vi "Dictionary ( Variant ).vi"() -> ()   [LabVIEW 2013]
panel:
  out "values":variant[](array[variant])
  out "names":string[](array[string])
  out "variant out":variant
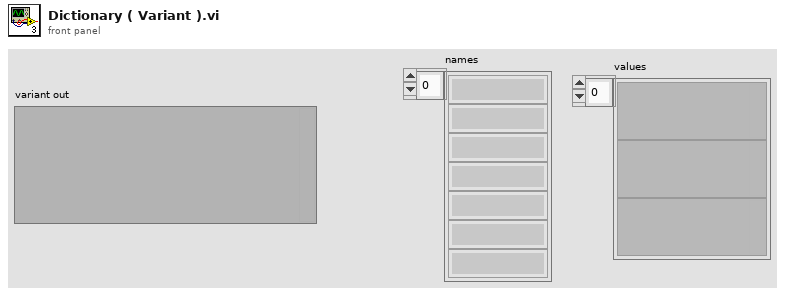
[diagram p1: front panel]
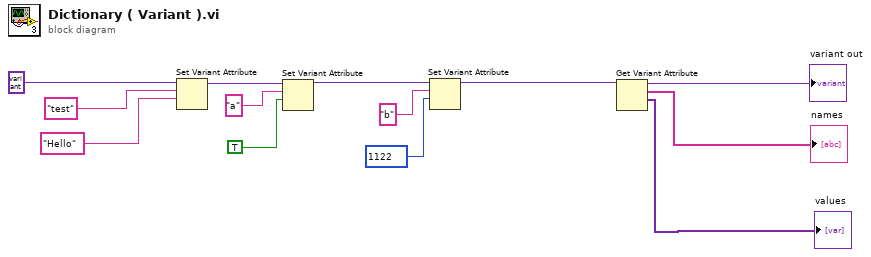
[diagram p0: block diagram]
diagram:
  n1 = Set Variant Attribute(Variant=variant ("variant"), name="test", value="Hello" ("name")) -> (Variant out=w8:variant)  [unwired: 1 in, 2 out]
  n2 = Set Variant Attribute(Variant=w8, name="a", value=TRUE) -> (Variant out=w4:variant)  [unwired: 1 in, 2 out]
  n3 = Set Variant Attribute(Variant=w4, name="b", value=1122) -> (Variant out=w3:variant)  [unwired: 1 in, 2 out]
  n4 = Get Variant Attribute(Variant=w3) -> (duplicate Variant=→"variant out":variant, names=→"names":string[], values=→"values":variant[])  [unwired: 3 in, 1 out]
